vi "LabelGrayImg.vi"(4 "Operation":T1(ring), 6 "Connectivity":bool, 8 "EorIn":errorcluster, 9 "Threshold Values":T3(slide)={"Minimum Value"=0.0, "Maximum Value"=65.106384} scale=0.0..255.0, 10 "Dst":T2(plugin-control), 11 "Src":T2(plugin-control)) -> (0 "ErrOut":errorcluster, 2 "# of Particles found":i32, 3 "ImgOut":T2(plugin-control))   [LabVIEW 2016]
doc: "Use this template to build a VI to use as a subVI."
uses:
  <vilib>/vision/NI_Vision_Development_Module.lvlib
panel:
  # "Output Parameters"
  # "Input Parameters"
  # "VI Description:\nThis VI is .."
  # ":: MVi Framework V1.0 ::\nAuthor:Gaoke Yang\nEmail: gaoke.yang@yahoo.com\nWeb: www.mvicontrol.com\nCopyright (C) 2015, MVI Technologies All Rights Reserved"
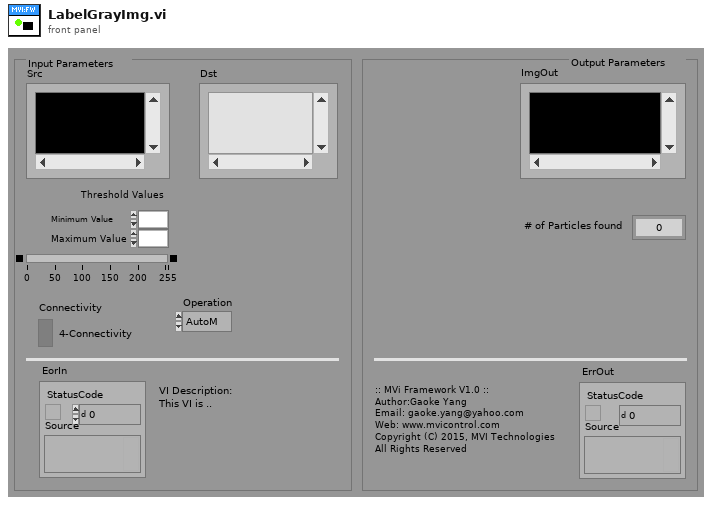
[diagram p1: front panel]
types:
  T1 = enum32{"AutoM", "Close", "Dilate", "Erode", "Gradient", "Gradient out", "Gradient in", "Hit miss", "Open", "PClose", "POpen", "Thick", "Thin"}
  T2 = typedef "IMAQ Image.ctl" = refnum<image>
  T3 = cluster{"Minimum Value":sgl, "Maximum Value":sgl}
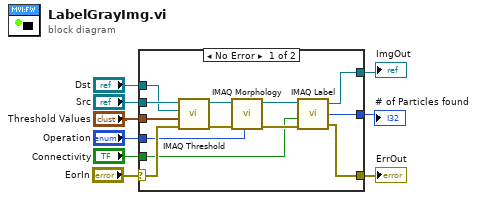
[diagram p0: block diagram]
diagram:
  n1 = case shown="No Error" "EorIn" {
    selector: "EorIn" -> [w18 w24]
    tunnel: [w11 w24] -> w8
    tunnel: [w14 w23] -> w6
    tunnel: "Src" -> [w15 w23]
    tunnel: "Threshold Values" -> [w17 _]
    tunnel: "Connectivity" -> [w16 _]
    tunnel: "Dst" -> [w13 _]
    tunnel: "Operation" -> [w12 _]
    tunnel: [w10 _] -> w1
    frame No Error {
      n2 = call "IMAQ Threshold"("error in (no error)"=w18, "Range"=w17, "Image Dst"=w13, "Image Src"=w15) -> ("error out"=w20:errorcluster, "Image Dst Out"=w22:T2)  [unwired: 6 in]
      n3 = call "IMAQ Morphology"("error in (no error)"=w20, "Operation"=w12, "Image Src"=w22) -> ("error out"=w19:errorcluster, "Image Dst Out"=w21:T2)  [unwired: 7 in]
      n4 = call "IMAQ Label"("error in (no error)"=w19, "Connectivity 4/8 (8)"=w16, "Image Src"=w21) -> ("error out"=w11:errorcluster, "Number of Particles"=w10:i32, "Image Dst Out"=w14:T2)  [unwired: 1 in]
    }
    frame Error {
    }
  }
  "ErrOut" <- w8
  "ImgOut" <- w6
  "# of Particles found" <- w1
